vi "SQL_Table_Unit_Test_Drive_System_insert.vi"(10 "时间标识":timestamp, 11 "动力子系统数据":T1) -> (3 "error out":errorcluster)   [LabVIEW 2014]
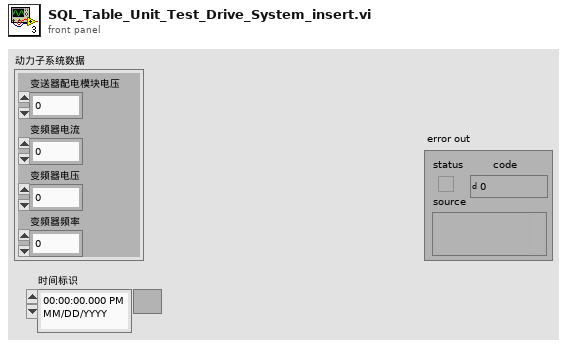
[diagram p1: front panel]
types:
  T1 = cluster{"变送器配电模块电压":u16, "变频器电流":u16, "变频器电压":u16, "变频器频率":u16}
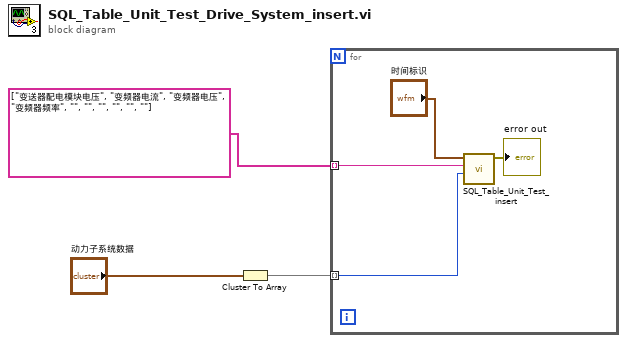
[diagram p0: block diagram]
diagram:
  n1 = Cluster To Array(cluster="动力子系统数据") -> (array=w2:u16[])
  n2 = for {
    tunnel: w2 -> [w6] mode=indexing
    tunnel: string[] ["变送器配电模块电压", "变频器电流", "变频器电压", "变频器频率", "", "", "", "", "", ""] -> [w5] mode=indexing
    n3 = call "SQL_Table_Unit_Test_insert.vi"("数据数值"=w6, "数据名称"=w5, "时间标识"="时间标识") -> ("error out"=→"error out":errorcluster)  [unwired: 8 in]
  }
